vi "Find Event Data.vi"(4 "Lower Sensor":dbl, 6 "Upper Sensor":dbl, 7 "Intensity Plot Ref":refnum<vi>, 8 "Event Name":u16, 9 "Backward":bool, 10 "Forward":bool, 11 "Data Cluster In":T1={"Selected File"=path "", "Full Text File"=[], "Data Array"=[], "Times Array"=[], "Sensor Array"=[], "Subset Array"=[], "Smoothness Values"=[], "Sensor Select 1"=refnum, "Sensor Select 2"=refnum, "Sensor Select 3"=refnum, "Sensor Select 4"=refnum, "Start Times"=[], "End Times"=[], "Cursor List"=[{"Name"="Event Marker          ", "Color"=16777200, "Style"=0, "Point Style"=0, "Name Visible"=FALSE, "Allow Drag"=FALSE, "Cursor Mode"=0, "Plot"=0, "Index"=0, "Position"={"X"=4.0, "Y"=1.0}, "X Scale"=0, "Y Scale"=0, "Watch Plots"=[], "Watch All Plots"=FALSE, "Plot Area"=0, "Label Offset"={"X"=-50.0, "Y"=150.0}}, {"Name"="Upper Sensor", "Color"=13816500, "Style"=6, "Point Style"=0, "Name Visible"=FALSE, "Allow Drag"=FALSE, "Cursor Mode"=0, "Plot"=0, "Index"=0, "Position"={"X"=-1.0, "Y"=5.0}, "X Scale"=0, "Y Scale"=0, "Watch Plots"=[], "Watch All Plots"=FALSE, "Plot Area"=0, "Label Offset"={"X"=0.0, "Y"=0.0}}, {"Name"="Lower Sensor", "Color"=13816500, "Style"=6, "Point Style"=0, "Name Visible"=FALSE, "Allow Drag"=FALSE, "Cursor Mode"=0, "Plot"=0, "Index"=0, "Position"={"X"=-1.0, "Y"=30.0}, "X Scale"=0, "Y Scale"=0, "Watch Plots"=[], "Watch All Plots"=FALSE, "Plot Area"=0, "Label Offset"={"X"=0.0, "Y"=0.0}}], "Listbox 1"=refnum, "Listbox 2"=refnum, "Listbox 3"=refnum, "Listbox 4"=refnum, "Labels"=["Why", "is", "this", "still", "not", "built", "into", "Labview?", "This", "is", "shameful."], "Event Array"=[], "Event Names"=[], "Event Times"=[], "Save Plot Button"=refnum, "Sensor Plot Refs"=[], "Selected Event (Title)"="", "Upper Cursor"=0.0, "Lower Cursor"=0.0, "Z Max"=0.0, "Z Min"=0.0}) -> (2 "Event Data Array":dbl[][](array[numeric]), 3 "output cluster":T1={"Selected File"=path "", "Full Text File"=[], "Data Array"=[], "Times Array"=[], "Sensor Array"=[], "Subset Array"=[], "Smoothness Values"=[], "Sensor Select 1"=refnum, "Sensor Select 2"=refnum, "Sensor Select 3"=refnum, "Sensor Select 4"=refnum, "Start Times"=[], "End Times"=[], "Cursor List"=[{"Name"="Event Marker          ", "Color"=16777200, "Style"=0, "Point Style"=0, "Name Visible"=FALSE, "Allow Drag"=FALSE, "Cursor Mode"=0, "Plot"=0, "Index"=0, "Position"={"X"=4.0, "Y"=1.0}, "X Scale"=0, "Y Scale"=0, "Watch Plots"=[], "Watch All Plots"=FALSE, "Plot Area"=0, "Label Offset"={"X"=-50.0, "Y"=150.0}}, {"Name"="Upper Sensor", "Color"=13816500, "Style"=6, "Point Style"=0, "Name Visible"=FALSE, "Allow Drag"=FALSE, "Cursor Mode"=0, "Plot"=0, "Index"=0, "Position"={"X"=-1.0, "Y"=5.0}, "X Scale"=0, "Y Scale"=0, "Watch Plots"=[], "Watch All Plots"=FALSE, "Plot Area"=0, "Label Offset"={"X"=0.0, "Y"=0.0}}, {"Name"="Lower Sensor", "Color"=13816500, "Style"=6, "Point Style"=0, "Name Visible"=FALSE, "Allow Drag"=FALSE, "Cursor Mode"=0, "Plot"=0, "Index"=0, "Position"={"X"=-1.0, "Y"=30.0}, "X Scale"=0, "Y Scale"=0, "Watch Plots"=[], "Watch All Plots"=FALSE, "Plot Area"=0, "Label Offset"={"X"=0.0, "Y"=0.0}}], "Listbox 1"=refnum, "Listbox 2"=refnum, "Listbox 3"=refnum, "Listbox 4"=refnum, "Labels"=["Why", "is", "this", "still", "not", "built", "into", "Labview?", "This", "is", "shameful."], "Event Array"=[], "Event Names"=[], "Event Times"=[], "Save Plot Button"=refnum, "Sensor Plot Refs"=[], "Selected Event (Title)"="", "Upper Cursor"=0.0, "Lower Cursor"=0.0, "Z Max"=0.0, "Z Min"=0.0})   [LabVIEW 2020]
uses:
  Controls/DataCluster.ctl
  <vilib>/Utility/miscctls.llb/LVCursorListTypeDef.ctl
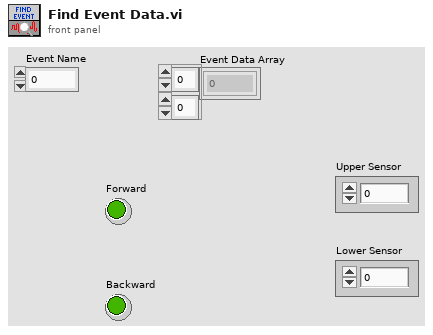
[diagram p1: front panel]
types:
  T1 = typedef "DataCluster.ctl" = cluster{"Selected File":path, "Full Text File":string[][], "Data Array":dbl[][], "Times Array":dbl[], "Sensor Array":dbl[], "Subset Array":dbl[][], "Smoothness Values":dbl[], "Sensor Select 1":refnum<vi>, "Sensor Select 2":refnum<vi>, "Sensor Select 3":refnum<vi>, "Sensor Select 4":refnum<vi>, "Start Times":dbl[], "End Times":dbl[], "Cursor List":T2, "Listbox 1":refnum<vi>, "Listbox 2":refnum<vi>, "Listbox 3":refnum<vi>, "Listbox 4":refnum<vi>, "Labels":string[], "Event Array":dbl[][], "Event Names":string[], "Event Times":dbl[], "Save Plot Button":refnum<vi>, "Sensor Plot Refs":refnum<vi>[], "Selected Event (Title)":string, "Upper Cursor":dbl, "Lower Cursor":dbl, "Z Max":dbl, "Z Min":dbl}
  T2 = typedef "LVCursorListTypeDef.ctl" = cluster{"Name":string, "Color":u32, "Style":u8, "Point Style":u8, "Name Visible":bool, "Allow Drag":bool, "Cursor Mode":u32, "Plot":i32, "Index":i32, "Position":cluster{"X":dbl, "Y":dbl}, "X Scale":u32, "Y Scale":u32, "Watch Plots":i32[], "Watch All Plots":bool, "Plot Area":i32, "Label Offset":cluster{"X":dbl, "Y":dbl}}[]
  T3 = cluster{"Cursor List[0]":cluster{"Name":string, "Color":u32, "Style":u8, "Point Style":u8, "Name Visible":bool, "Allow Drag":bool, "Cursor Mode":u32, "Plot":i32, "Index":i32, "Position":cluster{"X":dbl, "Y":dbl}, "X Scale":u32, "Y Scale":u32, "Watch Plots":i32[], "Watch All Plots":bool, "Plot Area":i32, "Label Offset":cluster{"X":dbl, "Y":dbl}}, "Cursor List[1]":cluster{"Name":string, "Color":u32, "Style":u8, "Point Style":u8, "Name Visible":bool, "Allow Drag":bool, "Cursor Mode":u32, "Plot":i32, "Index":i32, "Position":cluster{"X":dbl, "Y":dbl}, "X Scale":u32, "Y Scale":u32, "Watch Plots":i32[], "Watch All Plots":bool, "Plot Area":i32, "Label Offset":cluster{"X":dbl, "Y":dbl}}, "Cursor List[2]":cluster{"Name":string, "Color":u32, "Style":u8, "Point Style":u8, "Name Visible":bool, "Allow Drag":bool, "Cursor Mode":u32, "Plot":i32, "Index":i32, "Position":cluster{"X":dbl, "Y":dbl}, "X Scale":u32, "Y Scale":u32, "Watch Plots":i32[], "Watch All Plots":bool, "Plot Area":i32, "Label Offset":cluster{"X":dbl, "Y":dbl}}, "Cursor List[3]":cluster{"Name":string, "Color":u32, "Style":u8, "Point Style":u8, "Name Visible":bool, "Allow Drag":bool, "Cursor Mode":u32, "Plot":i32, "Index":i32, "Position":cluster{"X":dbl, "Y":dbl}, "X Scale":u32, "Y Scale":u32, "Watch Plots":i32[], "Watch All Plots":bool, "Plot Area":i32, "Label Offset":cluster{"X":dbl, "Y":dbl}}, "Cursor List[4]":cluster{"Name":string, "Color":u32, "Style":u8, "Point Style":u8, "Name Visible":bool, "Allow Drag":bool, "Cursor Mode":u32, "Plot":i32, "Index":i32, "Position":cluster{"X":dbl, "Y":dbl}, "X Scale":u32, "Y Scale":u32, "Watch Plots":i32[], "Watch All Plots":bool, "Plot Area":i32, "Label Offset":cluster{"X":dbl, "Y":dbl}}, "Cursor List[5]":cluster{"Name":string, "Color":u32, "Style":u8, "Point Style":u8, "Name Visible":bool, "Allow Drag":bool, "Cursor Mode":u32, "Plot":i32, "Index":i32, "Position":cluster{"X":dbl, "Y":dbl}, "X Scale":u32, "Y Scale":u32, "Watch Plots":i32[], "Watch All Plots":bool, "Plot Area":i32, "Label Offset":cluster{"X":dbl, "Y":dbl}}, "Cursor List[6]":cluster{"Name":string, "Color":u32, "Style":u8, "Point Style":u8, "Name Visible":bool, "Allow Drag":bool, "Cursor Mode":u32, "Plot":i32, "Index":i32, "Position":cluster{"X":dbl, "Y":dbl}, "X Scale":u32, "Y Scale":u32, "Watch Plots":i32[], "Watch All Plots":bool, "Plot Area":i32, "Label Offset":cluster{"X":dbl, "Y":dbl}}, "Cursor List[7]":cluster{"Name":string, "Color":u32, "Style":u8, "Point Style":u8, "Name Visible":bool, "Allow Drag":bool, "Cursor Mode":u32, "Plot":i32, "Index":i32, "Position":cluster{"X":dbl, "Y":dbl}, "X Scale":u32, "Y Scale":u32, "Watch Plots":i32[], "Watch All Plots":bool, "Plot Area":i32, "Label Offset":cluster{"X":dbl, "Y":dbl}}, "Cursor List[8]":cluster{"Name":string, "Color":u32, "Style":u8, "Point Style":u8, "Name Visible":bool, "Allow Drag":bool, "Cursor Mode":u32, "Plot":i32, "Index":i32, "Position":cluster{"X":dbl, "Y":dbl}, "X Scale":u32, "Y Scale":u32, "Watch Plots":i32[], "Watch All Plots":bool, "Plot Area":i32, "Label Offset":cluster{"X":dbl, "Y":dbl}}}
  T4 = cluster{"Name":string, "Color":u32, "Style":u8, "Point Style":u8, "Name Visible":bool, "Allow Drag":bool, "Cursor Mode":u32, "Plot":i32, "Index":i32, "Position":cluster{"X":dbl, "Y":dbl}, "X Scale":u32, "Y Scale":u32, "Watch Plots":i32[], "Watch All Plots":bool, "Plot Area":i32, "Label Offset":cluster{"X":dbl, "Y":dbl}}[]
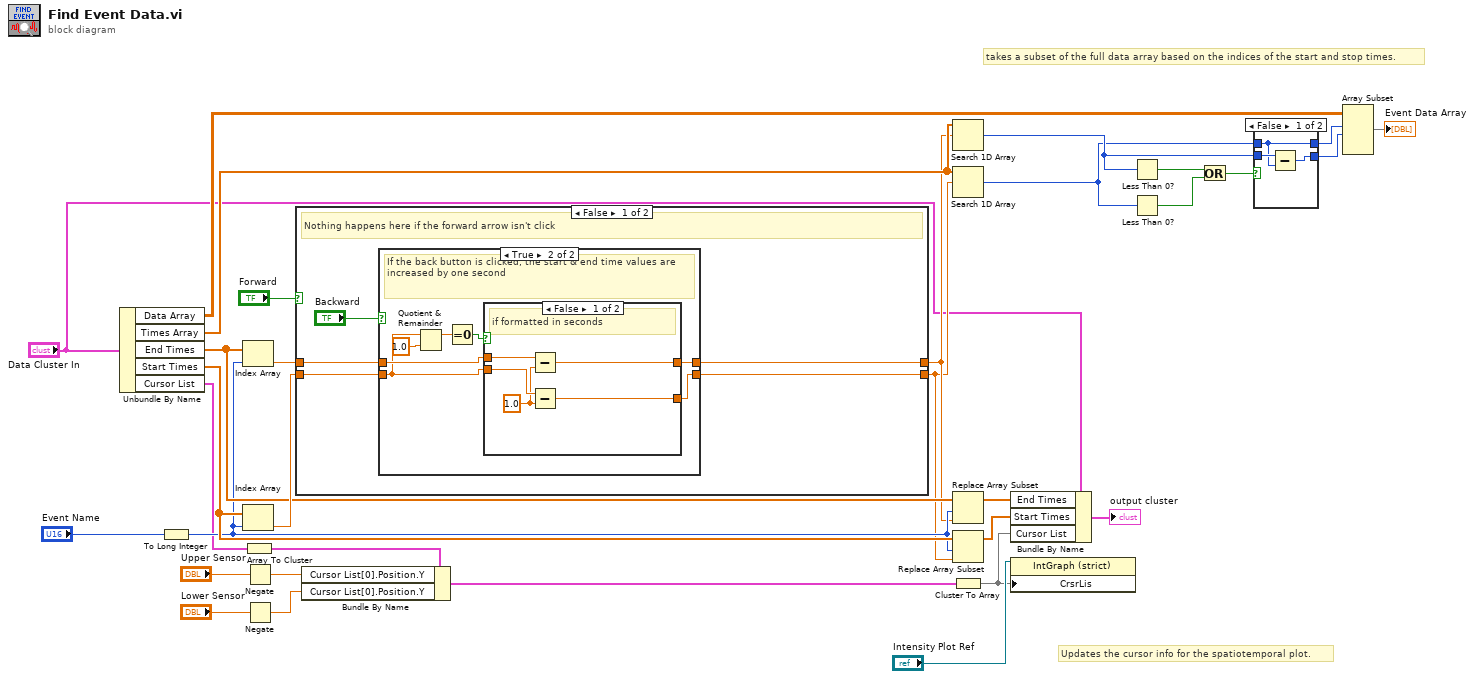
[diagram p0: block diagram]
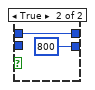
[diagram p2: hidden frame]
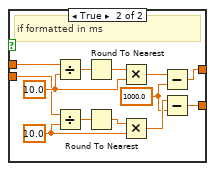
[diagram p4: hidden frame]
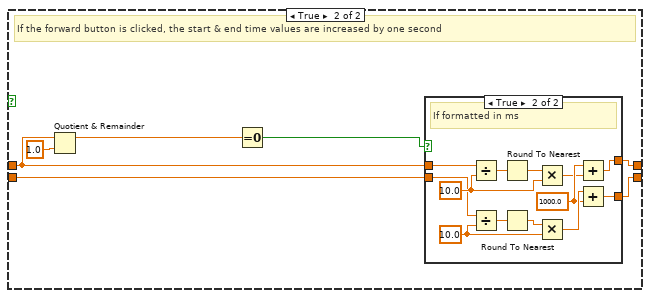
[diagram p5: hidden frame]
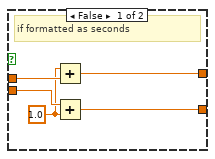
[diagram p6: hidden frame]
diagram:
  # "takes a subset of the full data array based on the indices of the start and stop times."
  # "Updates the cursor info for the spatiotemporal plot."
  n1 = Unbundle By Name("Data Cluster In") -> ("Data Array"=w27:dbl[][], "Times Array"=w26:dbl[], "End Times"=w25:dbl[], "Start Times"=w24:dbl[], "Cursor List"=w18:T2)
  n2 = To Long Integer(number="Event Name") -> (32bit integer=w23:i32)
  n3 = Index Array(array=w25, index=w23) -> (element=w28:dbl)
  n4 = Index Array(array=w24, index=w23) -> (element=w29:dbl)
  n5 = Array To Cluster(array=w18) -> (cluster=w4:T3)
  n6 = Negate(x="Upper Sensor") -> (-x=w14:dbl)
  n7 = Negate(x="Lower Sensor") -> (-x=w13:dbl)
  n8 = case shown="False" "Forward" {
    tunnel: [w33 w68] -> w19
    tunnel: [w34 w67] -> w20
    tunnel: w29 -> [w37 w66]
    tunnel: w28 -> [w36 w65]
    frame False {
      # "Nothing happens here if the forward arrow isn't click"
      n9 = case shown="True" "Backward" {
        tunnel: w37 -> [w38 w40]
        tunnel: w36 -> [w39 w46]
        tunnel: [w38 w43] -> w33
        tunnel: [w39 w42] -> w34
        frame False {
        }
        frame True {
          # "If the back button is clicked, the start & end time values are increased by one second"
          n10 = Quotient & Remainder(x=w40, y=1.0) -> (x-y*floor(x/y)=w41:dbl)  [unwired: 1 out]
          n11 = Equal To 0?(x=w41) -> (x = 0?=w44:bool)
          n12 = case shown="False" w44 {
            tunnel: [w49 w55] -> w42
            tunnel: w40 -> [w51 w58]
            tunnel: [w50 w56] -> w43
            tunnel: w46 -> [w48 w52]
            frame False {
              w47 = 1.0 ("y")
              # "if formatted in seconds"
              n13 = Subtract(x=w48, y=w47) -> (x-y=w49:dbl)
              n14 = Subtract(x=w51, y=w47) -> (x-y=w50:dbl)
            }
            frame True {
              w59 = 10.0 ("y")
              w53 = 1000.0 ("y")
              w62 = 10.0 ("y")
              # "if formatted in ms"
              n15 = Divide(x=w52, y=w62) -> (x/y=w63:dbl)
              n16 = Divide(x=w58, y=w59) -> (x/y=w60:dbl)
              n17 = Round To Nearest(number=w63) -> (nearest integer value=w64:dbl)
              n18 = Round To Nearest(number=w60) -> (nearest integer value=w61:dbl)
              n19 = Multiply(x=w64, y=w62) -> (x*y=w54:dbl)
              n20 = Multiply(x=w61, y=w59) -> (x*y=w57:dbl)
              n21 = Subtract(x=w54, y=w53) -> (x-y=w55:dbl)
              n22 = Subtract(x=w57, y=w53) -> (x-y=w56:dbl)
            }
          }
        }
      }
    }
    frame True {
      # "If the forward button is clicked, the start & end time values are increased by one second"
      n23 = Quotient & Remainder(x=w65, y=1.0) -> (x-y*floor(x/y)=w70:dbl)  [unwired: 1 out]
      n24 = Equal To 0?(x=w70) -> (x = 0?=w69:bool)
      n25 = case shown="True" w69 {
        tunnel: [w72 w77] -> w67
        tunnel: w65 -> [w75 w86]
        tunnel: w66 -> [w76 w82]
        tunnel: [w73 w80] -> w68
        frame False {
          w74 = 1.0 ("y")
          # "if formatted as seconds"
          n26 = Add(x=w74, y=w75) -> (x+y=w72:dbl)
          n27 = Add(x=w76, y=w74) -> (x+y=w73:dbl)
        }
        frame True {
          w83 = 10.0 ("y")
          w79 = 1000.0 ("y")
          w87 = 10.0 ("y")
          # "If formatted in ms"
          n28 = Divide(x=w86, y=w87) -> (x/y=w88:dbl)
          n29 = Divide(x=w82, y=w83) -> (x/y=w84:dbl)
          n30 = Round To Nearest(number=w88) -> (nearest integer value=w89:dbl)
          n31 = Round To Nearest(number=w84) -> (nearest integer value=w85:dbl)
          n32 = Multiply(x=w89, y=w87) -> (x*y=w78:dbl)
          n33 = Multiply(x=w85, y=w83) -> (x*y=w81:dbl)
          n34 = Add(x=w79, y=w78) -> (x+y=w77:dbl)
          n35 = Add(x=w81, y=w79) -> (x+y=w80:dbl)
        }
      }
    }
  }
  n36 = Bundle By Name(cluster=w4, "Cursor List[0].Position.Y"=w14, "Cursor List[0].Position.Y"=w13) -> (w15:T3)
  n37 = Search 1D Array(1D array=w26, element=w20) -> (index of element=w8:i32)  [unwired: 1 in]
  n38 = Search 1D Array(1D array=w26, element=w19) -> (index of element=w7:i32)  [unwired: 1 in]
  n39 = Replace Array Subset(array=w25, new element=w20, index=w23) -> (w21:dbl[])
  n40 = Replace Array Subset(array=w24, new element=w19, index=w23) -> (w22:dbl[])
  n41 = Cluster To Array(cluster=w15) -> (array=w2:T4)
  n42 = Bundle By Name(cluster="Data Cluster In", "End Times"=w21, "Start Times"=w22, "Cursor List"=w2) -> (→"output cluster":T1)
  n43 = property class="IntGraph (strict)"(reference="Intensity Plot Ref", "CrsrLis"=w2) -> ()  [unwired: 1 in, 2 out]
  n44 = Less Than 0?(x=w8) -> (x < 0?=w11:bool)
  n45 = Less Than 0?(x=w7) -> (x < 0?=w10:bool)
  n46 = Or(x=w11, y=w10) -> (x .or. y?=w9:bool)
  n47 = case shown="False" w9 {
    tunnel: w8 -> [w91 _]
    tunnel: w7 -> [w90 w93]
    tunnel: [w92 800] -> w6
    tunnel: [w90 w93] -> w5
    frame False {
      n48 = Subtract(x=w91, y=w90) -> (x-y=w92:i32)
    }
    frame True {
    }
  }
  n49 = Array Subset(array=w27, index (row)=w5, length (row)=w6) -> (→"Event Data Array":dbl[][])  [unwired: 2 in]
